vi "vertical spacing values.vi"() -> (2 "Section spacing":u32=15, 3 "Control spacing":u32=7)   [LabVIEW 2020, in "verticalDistribution.lvlib"]
uses:
  <vilib>/Utility/vertDist/verticalDistribution.lvlib
panel:
  # "Vertical spacing between controls"
  # "Vertical spacing before all sections\nexcept first section, which doesn't\nset any spacing before it."
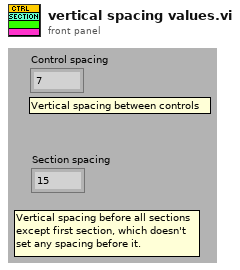
[diagram p1: front panel]
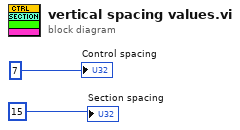
[diagram p0: block diagram]
diagram:
  "Control spacing" <- u32 7 ("Control spacing")
  "Section spacing" <- u32 15 ("Section spacing")
